vi "DisplacementASCIIDigitToNumber.vi"(11 "Value":u8) -> (2 "Number":i32, 3 "Valid":bool)   [LabVIEW 2016]
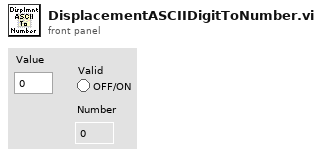
[diagram p1: front panel]
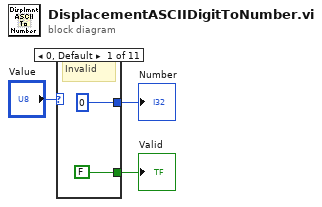
[diagram p0: block diagram]
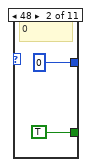
[diagram p2: hidden frame]
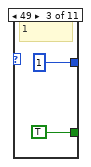
[diagram p3: hidden frame]
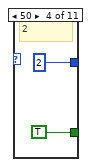
[diagram p4: hidden frame]
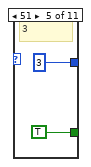
[diagram p5: hidden frame]
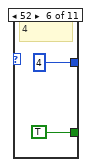
[diagram p6: hidden frame]
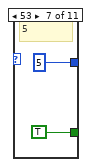
[diagram p7: hidden frame]
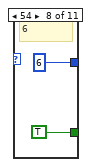
[diagram p8: hidden frame]
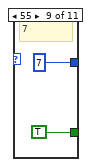
[diagram p9: hidden frame]
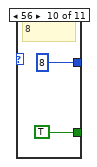
[diagram p10: hidden frame]
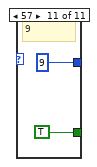
[diagram p11: hidden frame]
diagram:
  n1 = case shown="0, Default" "Value" {
    tunnel: [0 0 1 2 3 4 5 6 7 8 9] -> w2
    tunnel: [FALSE TRUE TRUE TRUE TRUE TRUE TRUE TRUE TRUE TRUE TRUE] -> w1
    frame 0, Default {
      # "Invalid"
    }
    frame 48 {
      # "0"
    }
    frame 49 {
      # "1"
    }
    frame 50 {
      # "2"
    }
    frame 51 {
      # "3"
    }
    frame 52 {
      # "4"
    }
    frame 53 {
      # "5"
    }
    frame 54 {
      # "6"
    }
    frame 55 {
      # "7"
    }
    frame 56 {
      # "8"
    }
    frame 57 {
      # "9"
    }
  }
  "Number" <- w2
  "Valid" <- w1
